vi "Slope Data Acquisition.vi"() -> (0 "Deviation Signal":dbl[](array[numeric]), 1 "Z Piezo Signal":dbl[](array[numeric]))   [LabVIEW 2013]
uses:
  <vilib>/DAQmx/write.llb/DAQmx Write (Analog 1D Wfm NChan NSamp).vi
  <vilib>/DAQmx/read.llb/DAQmx Read (Analog 2D DBL NChan NSamp).vi
  <vilib>/DAQmx/create/channels.llb/DAQmx Create Channel (AI-Voltage-Basic).vi
  <vilib>/DAQmx/create/channels.llb/DAQmx Create Channel (AO-Voltage-Basic).vi
  <vilib>/DAQmx/configure/timing.llb/DAQmx Timing (Use Waveform).vi
  <vilib>/DAQmx/configure/trigger.llb/DAQmx Start Trigger (Digital Edge).vi
  <vilib>/DAQmx/configure/timing.llb/DAQmx Timing (Sample Clock).vi
  <vilib>/DAQmx/miscellaneous.llb/DAQmx Fill In Error Info.vi
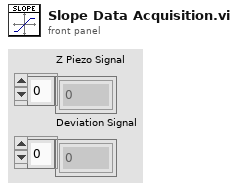
[diagram p1: front panel]
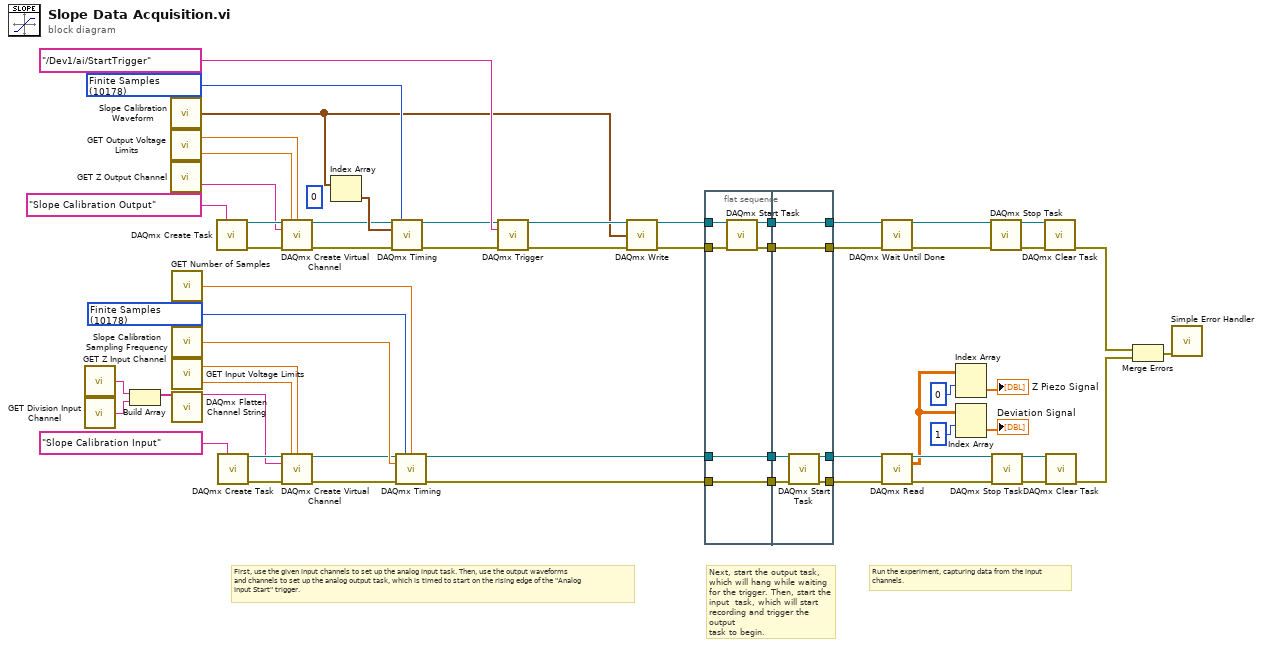
[diagram p0: block diagram]
diagram:
  w45 = 10178 items=["Finite Samples"=10178, "Continuous Samples"=10123, "Hardware Timed Single Point"=12522] ("sample mode")
  (unwired) 0 ("index")
  w35 = 10178 items=["Finite Samples"=10178, "Continuous Samples"=10123, "Hardware Timed Single Point"=12522] ("sample mode")
  # "Run the experiment, capturing data from the input \nchannels."
  # "Next, start the output task,\nwhich will hang while waiting\nfor the trigger. Then, start the\ninput  task, which will start \nrecording and trigger the output\ntask to begin."
  # "First, use the given input channels to set up the analog input task. Then, use the output waveforms\nand channels to set up the analog output task, which is timed to start on the rising edge of the \"Analog\nInput Start\" trigger."
  n1 = call "GET Z Input Channel.vi"() -> ("Z Input Channel"=w6:string)
  n2 = call "GET Division Input Channel.vi"() -> ("Division Input Channel"=w5:string)
  n3 = Build Array(w6, w5) -> (w4:string[])
  n4 = call "Slope Calibration Waveform.vi"() -> ("Slope Calibration Waveform"=w1:waveform(dbl)[])
  n5 = call "GET Output Voltage Limits.vi"() -> ("Maximum Output Voltage"=w51:dbl, "Minimum Output Voltage"=w52:dbl)
  n6 = call "GET Z Output Channel.vi"() -> ("Z Output Channel"=w2:string)
  n7 = call "GET Number of Samples.vi"() -> ("Number of Samples"=w46:dbl)
  n8 = call "Slope Calibration Sampling Frequency.vi"() -> ("Sampling Frequency"=w47:dbl)
  n9 = call "GET Input Voltage Limits.vi"() -> ("Maximum Input Voltage"=w49:dbl, "Minimum Input Voltage"=w50:dbl)
  n10 = call <vilib>:"DAQmx Flatten Channel String.vi"("names in"=w4) -> ("names out"=w3:string)  [unwired: 13 in, 1 out]
  n11 = call <vilib>:"DAQmx Create Task.vi"("new task name"="Slope Calibration Output") -> ("task out"=w30:refnum<k21>, "error out"=w24:errorcluster)  [unwired: 13 in]
  n12 = call <vilib>:"DAQmx Create Task.vi"("new task name"="Slope Calibration Input") -> ("task out"=w38:refnum<k21>, "error out"=w39:errorcluster)  [unwired: 13 in]
  n13 = call-poly <vilib>:"DAQmx Create Virtual Channel.vi"("task in"=w30, "maximum value"=w51, "minimum value"=w52, "physical channels"=w2, "error in"=w24) -> ("task out"=w31:refnum<k21>, "error out"=w25:errorcluster)  [unwired: 9 in]
  n14 = call-poly <vilib>:"DAQmx Create Virtual Channel.vi"("task in"=w38, "maximum value"=w49, "minimum value"=w50, "physical channels"=w3, "error in"=w39) -> ("task out"=w40:refnum<k21>, "error out"=w41:errorcluster)  [unwired: 9 in]
  n15 = Index Array(array=w1) -> (element=w36:waveform(dbl))  [unwired: 1 in]
  n16 = call-poly <vilib>:"DAQmx Timing.vi"("task/channels in"=w31, "sample mode"=w35, "waveform"=w36, "error in"=w25) -> ("task out"=w32:refnum<k21>, "error out"=w26:errorcluster)  [unwired: 10 in]
  n17 = call-poly <vilib>:"DAQmx Timing.vi"("task/channels in"=w40, "sample mode"=w45, "samples per channel"=w46, "rate"=w47, "error in"=w41) -> ("task out"=w42:refnum<k21>, "error out"=w43:errorcluster)  [unwired: 9 in]
  n18 = call-poly <vilib>:"DAQmx Trigger.vi"("task/channels in"=w32, "source"=tag "/Dev1/ai/StartTrigger" ("DAQmx Terminal"), "error in"=w26) -> ("task out"=w33:refnum<k21>, "error out"=w27:errorcluster)  [unwired: 11 in]
  n19 = call-poly <vilib>:"DAQmx Write.vi"("task/channels in"=w33, "data"=w1, "error in"=w27) -> ("task out"=w29:refnum<k21>, "error out"=w28:errorcluster)  [unwired: 10 in, 1 out]
  n20 = flat-sequence {
    tunnel: w28 -> [w62]
    tunnel: w29 -> [w60]
    tunnel: [w61] -> w56
    tunnel: [w59] -> w55
    tunnel: [w58] -> w54
    tunnel: w42 -> [w58]
    tunnel: [w57] -> w53
    tunnel: w43 -> [w57]
    tunnel: w56 -> [w66]
    tunnel: w55 -> [w65]
    tunnel: w54 -> [w68]
    tunnel: w53 -> [w67]
    tunnel: [w66] -> w11
    tunnel: [w65] -> w10
    tunnel: [w64] -> w9
    tunnel: [w63] -> w8
    frame #0 {
      n21 = call <vilib>:"DAQmx Start Task.vi"("task/channels in"=w60, "error in"=w62) -> ("task out"=w59:refnum<k21>, "error out"=w61:errorcluster)  [unwired: 12 in]
    }
    frame #1 {
      n22 = call <vilib>:"DAQmx Start Task.vi"("task/channels in"=w68, "error in"=w67) -> ("task out"=w64:refnum<k21>, "error out"=w63:errorcluster)  [unwired: 12 in]
    }
  }
  n23 = call <vilib>:"DAQmx Wait Until Done.vi"("task/channels in"=w10) -> ("task out"=w12:refnum<k21>, "error out"=w13:errorcluster)  [unwired: 13 in]
  n24 = call-poly <vilib>:"DAQmx Read.vi"("task/channels in"=w9) -> ("task out"=w16:refnum<k21>, "data"=w7:dbl[][], "error out"=w17:errorcluster)  [unwired: 12 in]
  n25 = Index Array(array=w7, index (row)=0) -> (element=→"Z Piezo Signal":dbl[])  [unwired: 1 in]
  n26 = Index Array(array=w7, index (row)=1) -> (element=→"Deviation Signal":dbl[])  [unwired: 1 in]
  n27 = call <vilib>:"DAQmx Stop Task.vi"("task/channels in"=w12, "error in"=w13) -> ("task out"=w15:refnum<k21>, "error out"=w14:errorcluster)  [unwired: 12 in]
  n28 = call <vilib>:"DAQmx Stop Task.vi"("task/channels in"=w16, "error in"=w17) -> ("task out"=w18:refnum<k21>, "error out"=w19:errorcluster)  [unwired: 12 in]
  n29 = call <vilib>:"DAQmx Clear Task.vi"("task in"=w15, "error in"=w14) -> ()  [unwired: 13 in, 1 out]
  n30 = call <vilib>:"DAQmx Clear Task.vi"("task in"=w18, "error in"=w19) -> ()  [unwired: 13 in, 1 out]
  n31 = Merge Errors(w11, w8) -> (w48:errorcluster)
  n32 = call <vilib>:"Simple Error Handler.vi"("error in (no error)"=w48) -> ()  [unwired: 4 in, 5 out]
